vi "measure_voltage.vi"(5 "Filename":path=path "test.lvm", 7 "rate":dbl=100.0, 9 "number of samples":i32=100) -> (1 "data":dynamicdata(graph))   [LabVIEW 2017]
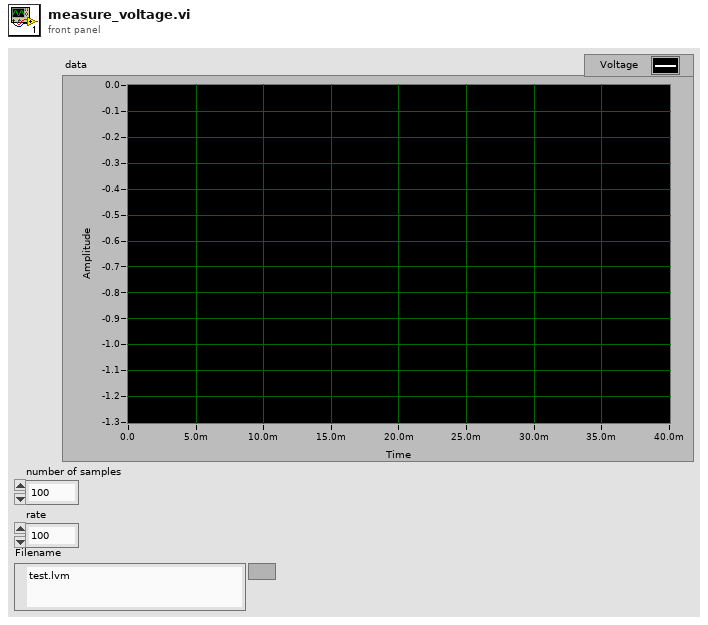
[diagram p1: front panel]
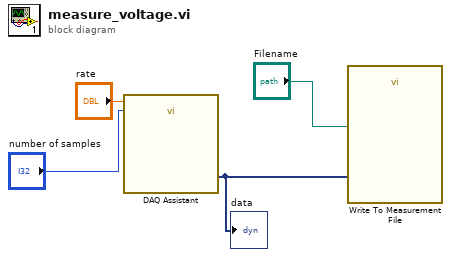
[diagram p0: block diagram]
diagram:
  n1 = call "DAQ Assistant"("rate"="rate", "number of samples"="number of samples") -> ("data"=w2:dynamicdata)  [unwired: 15 in, 2 out]
  "data" <- w2
  n2 = call "Write To Measurement File"("Signals"=w2, "Filename"="Filename") -> ()  [unwired: 15 in, 3 out]
